vi "getConfigFileSharedEnum.vi"() -> (3 "configFileSharedEnum":path)   [LabVIEW 2018]
doc: "Get the configuration file of shared enumeration."
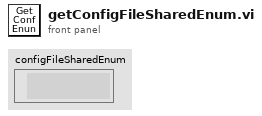
[diagram p1: front panel]
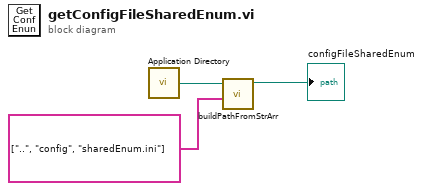
[diagram p0: block diagram]
diagram:
  n1 = call <vilib>:"Application Directory.vi"() -> ("Application Directory"=w3:path)
  n2 = call "buildPathFromStrArr.vi"("String Array"=string[] ["..", "config", "sharedEnum.ini"], "Root Path"=w3) -> ("Absolute Path"=→"configFileSharedEnum":path)  [unwired: 9 in]
